vi "Test Verify as JSON.vi"(11 "Test Case In":refnum<class "Core Library Error Propagation.lvclass">) -> (0 "error out":errorcluster, 3 "Test Case Out":refnum<class "Core Library Error Propagation.lvclass">)   [LabVIEW 2020, in "Core Library Error Propagation.lvclass"]
uses:
  Core Library Error Propagation.lvclass
  C:/Program Files/National Instruments/LabVIEW 2026/vi.lib/Astemes/LUnit/Test Case.lvclass
  Source/Approval Tests/Options/Options.lvclass
  <vilib>/Astemes/LUnit/Test Case.lvclass/Test Case.ctl
  <vilib>/Astemes/LUnit/Palette/Pass If Error.vi
  <vilib>/Astemes/LUnit/Palette/Advanced Assertions/Pass If Specific Error.vi/d0e67a5c-31db-4060-a993-98defbf94426.vi
  <vilib>/Astemes/LUnit/Palette/Fail.vi
  <vilib>/Astemes/LUnit/Core/LUnit Test Case/Private/Append Fail Result.vi
  <vilib>/Astemes/LUnit/Core/LUnit Test Case/Private/Append Pass Result.vi
  <vilib>/Astemes/LUnit/Core/LUnit Test Case/Private/Run In UI.vi
  <vilib>/Utility/error.llb/Clear Errors.vi
  <vilib>/Comparison/Equal/Equal Functor/Equal Functor.lvclass
  <vilib>/Astemes/LUnit/Palette/Advanced Assertions/LUnit Advanced Assertions.lvlib
  Source/Approval Tests/Approval Tests.lvlib
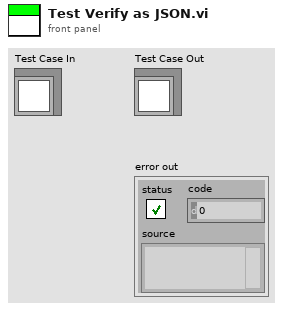
[diagram p1: front panel]
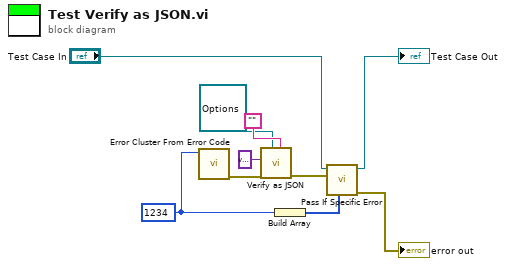
[diagram p0: block diagram]
diagram:
  w4 = 1234 ("error code (0)")
  n1 = call <vilib>:"Error Cluster From Error Code.vi"("error code (0)"=w4) -> ("error out"=w9:errorcluster)  [unwired: 8 in]
  n2 = call "Verify as JSON.vi"("Label"="", "Approval Tests.lvlib:Options.lvclass"=refnum<class "Options.lvclass"> refnum, "error in"=w9, "Anything"=variant) -> ("error out"=w8:errorcluster)  [unwired: 5 in, 2 out]
  n3 = Build Array(w4) -> (w5:i32[])
  n4 = call <vilib>:"Pass If Specific Error.vi"("Error Codes"=w5, "Assert error"=w8, "LUnit Test Case In"="Test Case In") -> ("error out"=→"error out":errorcluster, "LUnit Test Case Out"=→"Test Case Out":refnum<class "Core Library Error Propagation.lvclass">)  [unwired: 7 in]
